vi "lightsource-init.vi"(3 "error in 2":errorcluster, 5 "VISA in":refnum<visa-resource-name>="COM3") -> (0 "error out":errorcluster, 1 "initialized":bool=TRUE, 2 "VISA out":refnum<visa-resource-name>)   [LabVIEW 2017]
panel:
  in  "InParameters":T1={"Destination"=2, "Source"=162, "Register"=16, "Array"=[], "WriteNotRead"=FALSE, "ReadWithPreample"=FALSE, "Ring"=0, "String"="", "Long"=0} {"Ring" items=["ByteArray", "IntegerArray", "String", "Long", "Direct string sent"]; "Register" format="%x"}
  in  "PortParameters":T2={"OpenPort"=FALSE, "ClosePort"=FALSE, "Baudrate"=115200, "Wait"=50, "ReadWrite"=TRUE}
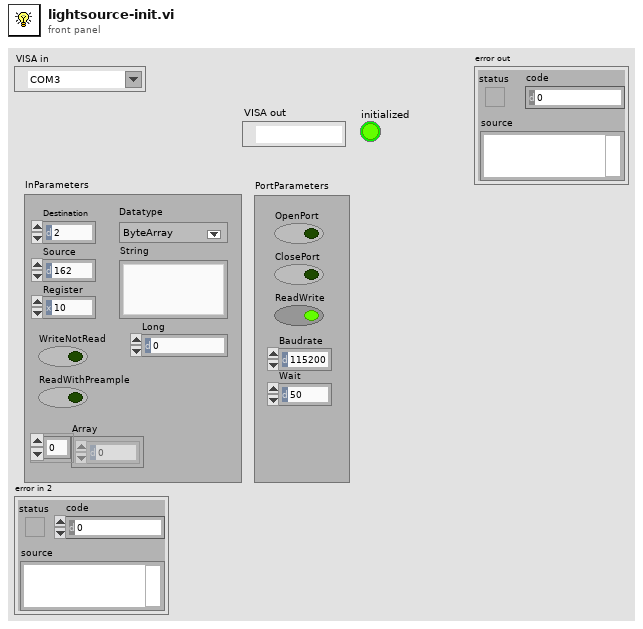
[diagram p1: front panel]
types:
  T1 = cluster{"Destination":u8, "Source":u8, "Register":u8, "Array":i16[], "WriteNotRead":bool, "ReadWithPreample":bool, "Ring":u16, "String":string, "Long":i32}
  T2 = cluster{"OpenPort":bool, "ClosePort":bool, "Baudrate":i32, "Wait":u16, "ReadWrite":bool}
  T3 = cluster{"Source":u8, "TelegramType":u8, "Register":u8, "Destination":u8, "TelegramReceived":bool, "CRC error":bool, "PayloadByteArray":u8[], "(hi.lo)":u16, "Crc16":u16, "Long":i32, "PayloadIntArray":u16[], "String":string}
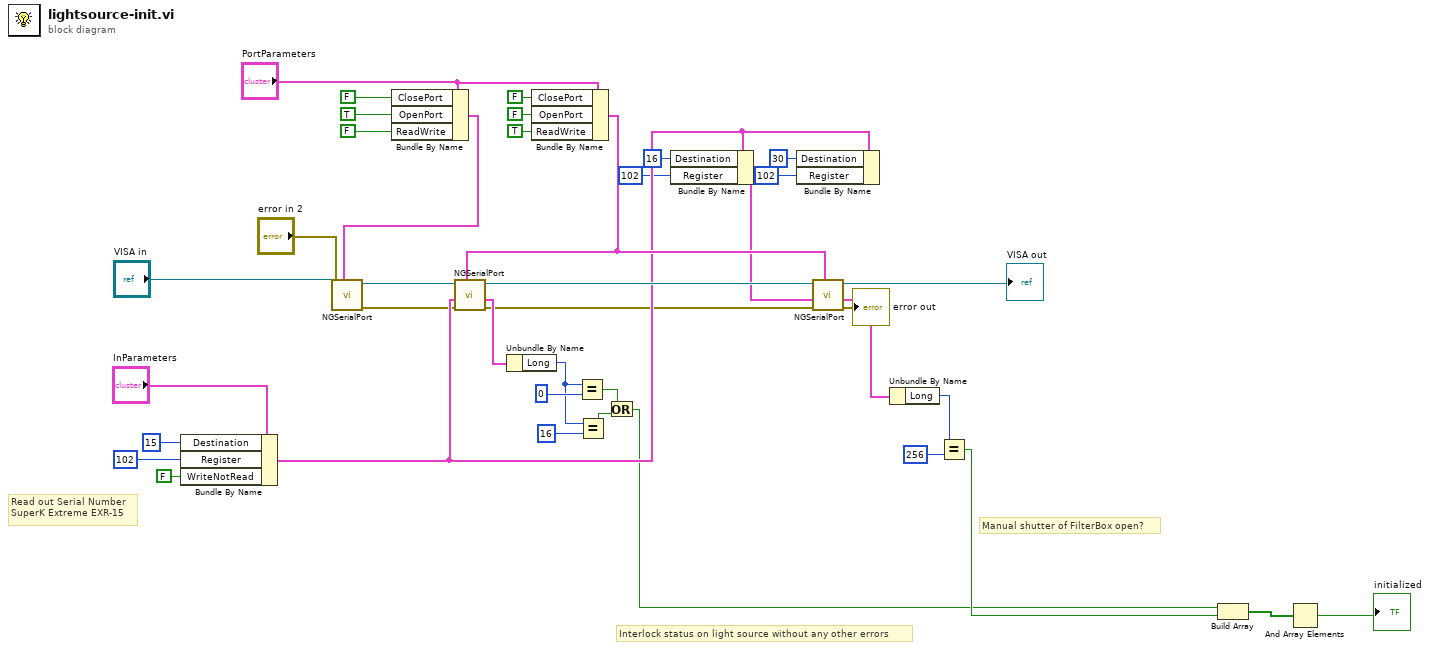
[diagram p0: block diagram]
diagram:
  # "Manual shutter of FilterBox open?"
  # "Interlock status on light source without any other errors"
  # "Read out Serial Number\nSuperK Extreme EXR-15"
  n1 = Bundle By Name(cluster="InParameters", "Destination"=u8 15, "Register"=u8 102, "WriteNotRead"=FALSE) -> (w22:T1)
  n2 = Bundle By Name(cluster="PortParameters", "ClosePort"=FALSE, "OpenPort"=TRUE, "ReadWrite"=FALSE) -> (w40:T2)
  n3 = call "NGSerialPort.vi"("PortParameters"=w40, "error in"="error in 2", "VISA in"="VISA in") -> ("error out"=w5:errorcluster, "VISA out"=w36:refnum<visa-resource-name>)  [unwired: 6 in, 1 out]
  n4 = Bundle By Name(cluster="PortParameters", "ClosePort"=FALSE, "OpenPort"=FALSE, "ReadWrite"=TRUE) -> (w24:T2)
  n5 = call "NGSerialPort.vi"("PortParameters"=w24, "error in"=w5, "InParameters"=w22, "VISA in"=w36) -> ("error out"=w4:errorcluster, "OutParameters"=w29:T3, "VISA out"=w28:refnum<visa-resource-name>)  [unwired: 5 in]
  n6 = Unbundle By Name(w29) -> ("Long"=w11:i32)
  n7 = Equal?(x=w11, y=0) -> (x = y?=w9:bool)
  n8 = Equal?(x=w11, y=16) -> (x = y?=w8:bool)
  n9 = Or(x=w9, y=w8) -> (x .or. y?=w7:bool)
  n10 = Bundle By Name(cluster=w22, "Destination"=u8 16, "Register"=u8 102) -> (w21:T1)
  n11 = Bundle By Name(cluster=w22, "Destination"=u8 30, "Register"=u8 102) -> ()  [unwired: 1 out]
  n12 = call "NGSerialPort.vi"("PortParameters"=w24, "error in"=w4, "InParameters"=w21, "VISA in"=w28) -> ("error out"=→"error out":errorcluster, "OutParameters"=w18:T3, "VISA out"=→"VISA out":refnum<visa-resource-name>)  [unwired: 5 in]
  n13 = Unbundle By Name(w18) -> ("Long"=w17:i32)
  n14 = Equal?(x=w17, y=256) -> (x = y?=w15:bool)
  n15 = Build Array(w7, w15) -> (w14:bool[])
  n16 = And Array Elements(Boolean array=w14) -> (logical AND=→"initialized":bool)
